vi "Robotics programming (Mohamed Elbakri 44171801).vi"() -> ()   [LabVIEW 2017]
uses:
  <vilib>/Native 3D Graph/xcontrol/3DPC_SurfacePlot.xctl
  <vilib>/Analysis/Matrix/Datatypes/RealMatrix.ctl
  <vilib>/Analysis/baseanly.llb/Real A x B.vi
  <vilib>/Analysis/baseanly.llb/Vector x A.vi
  <vilib>/Analysis/baseanly.llb/A x Vector.vi
  <vilib>/Analysis/NI_AALBase.lvlib
  <vilib>/Analysis/Matrix/NI_Matrix.lvlib
panel:
  in  "P2":dbl[](array[numeric])=[0.0, 0.0, 0.0]
  in  "P3":dbl[](array[numeric])=[0.0, 0.0, 0.0]
  in  "PE":dbl[](array[numeric])=[0.0, 0.0, 0.0]
  out "Out of range":bool
  out "?":dbl
  out "?":dbl
  out "PE":dbl[](array[numeric])
  out "P3":dbl[](array[numeric])
  out "P2":dbl[](array[numeric])
  out "b":dbl
  out "a":dbl
  out "T1":T1
  out "T2":T1
  out "T3":T1
  out "T1":T1
  out "T2":T1
  out "T3":T1
  out "T1":T1
  out "T2":T1
  out "T3":T1
  out "T1":T1
  out "T2":T1
  out "T3":T1
  in  "Z":dbl
  in  "Y":dbl
  in  "X":dbl
  in  "l0":dbl(slide) scale=0.0..10.0
  in  "l1":dbl(slide) scale=0.0..5.0
  in  "l2":dbl(slide) scale=0.0..5.0
  in  "l3":dbl(slide) scale=0.0..5.0
  out "Theta3":dbl(knob) scale=-90.0..90.0
  out "Theta2":dbl(knob) scale=-90.0..90.0
  out "Theta1":dbl(knob) scale=-180.0..180.0
  in  "Theta1":i16(knob) min=-180 max=180 step=1 scale=-180.0..180.0
  in  "Theta2":i8(knob) min=-90 max=90 step=1 scale=-90.0..90.0
  in  "Theta3":i8(knob) min=-90 max=90 step=1 scale=-90.0..90.0
  out "Control":dbl
  in  "Control":dbl=1.0 min=1.0 max=2.0 step=1.0
  out "S3":dbl(slide) scale=0.0..10.0
  out "S2":dbl(slide) scale=0.0..10.0
  out "S1":dbl(slide) scale=0.0..10.0
  in  "S3":i8(slide) scale=-10.0..10.0
  in  "S1":i8(slide) min=-10 max=10 step=1 scale=-10.0..10.0
  in  "S2":i8(slide) scale=-10.0..10.0
  in  "Robot":dbl=1.0 min=1.0 max=4.0 step=1.0 format="%#_4g"
  out "T3":T1
  out "T3":T1
  out "T3":T1
  out "T3":T1
  out "T1":T1
  out "T2":T1
  out "T1":T1
  out "T2":T1
  out "T1":T1
  out "T2":T1
  in  "stop":bool
  out "T2":T1
  out "T1":T1
  out "x_PE":dbl[](array[numeric])
  out "y_PE":dbl[](array[numeric])
  out "z_PE":dbl[](array[numeric])
  out "x_P3":dbl[](array[numeric])
  out "y_P3":dbl[](array[numeric])
  out "z_P3":dbl[](array[numeric])
  out "x_P2":dbl[](array[numeric])
  out "y_P2":dbl[](array[numeric])
  out "z_P2":dbl[](array[numeric])
  out "x_P1":dbl[](array[numeric])
  out "y_P1":dbl[](array[numeric])
  out "z_P1":dbl[](array[numeric])
  out "z_P0":dbl[](array[numeric])
  out "y_P0":dbl[](array[numeric])
  out "x_P0":dbl[](array[numeric])
  out "3D Graph":refnum<class "Base Datatype.lvclass">[](xcontrol)
  # "Robot Configuration"
  # "PE"
  # "Initial length"
  # "Joints position"
  # "L3"
  # "P3"
  # "L2"
  # "P2"
  # "L1"
  # "P1"
  # "L0"
  # "Control panel"
  # "Forward control"
  # "Joints control"
  # "Inverse control"
  # "Cartesian robot"
  # "Cylinderical robot"
  # "Spherical robot"
  # "Articulated robot"
  # "End-tip position"
  # "1: Cartesian robot"
  # "S3"
  # "L3"
  # "S3"
  # "2: Cylinderical robot"
  # "S3"
  # "Theta3"
  # "3: Spherical robot"
  # "L2"
  # "L2"
  # "4: Articulated robot"
  # "S2"
  # "Theta2"
  # "S2"
  # "Theta2"
  # "L1"
  # "L1"
  # "L1"
  # "Theta1"
  # "Theta1"
  # "S1"
  # "Theta1"
  # "1: Forward control"
  # "L0"
  # "L0"
  # "L0"
  # "2: Inverse control"
  # "L0"
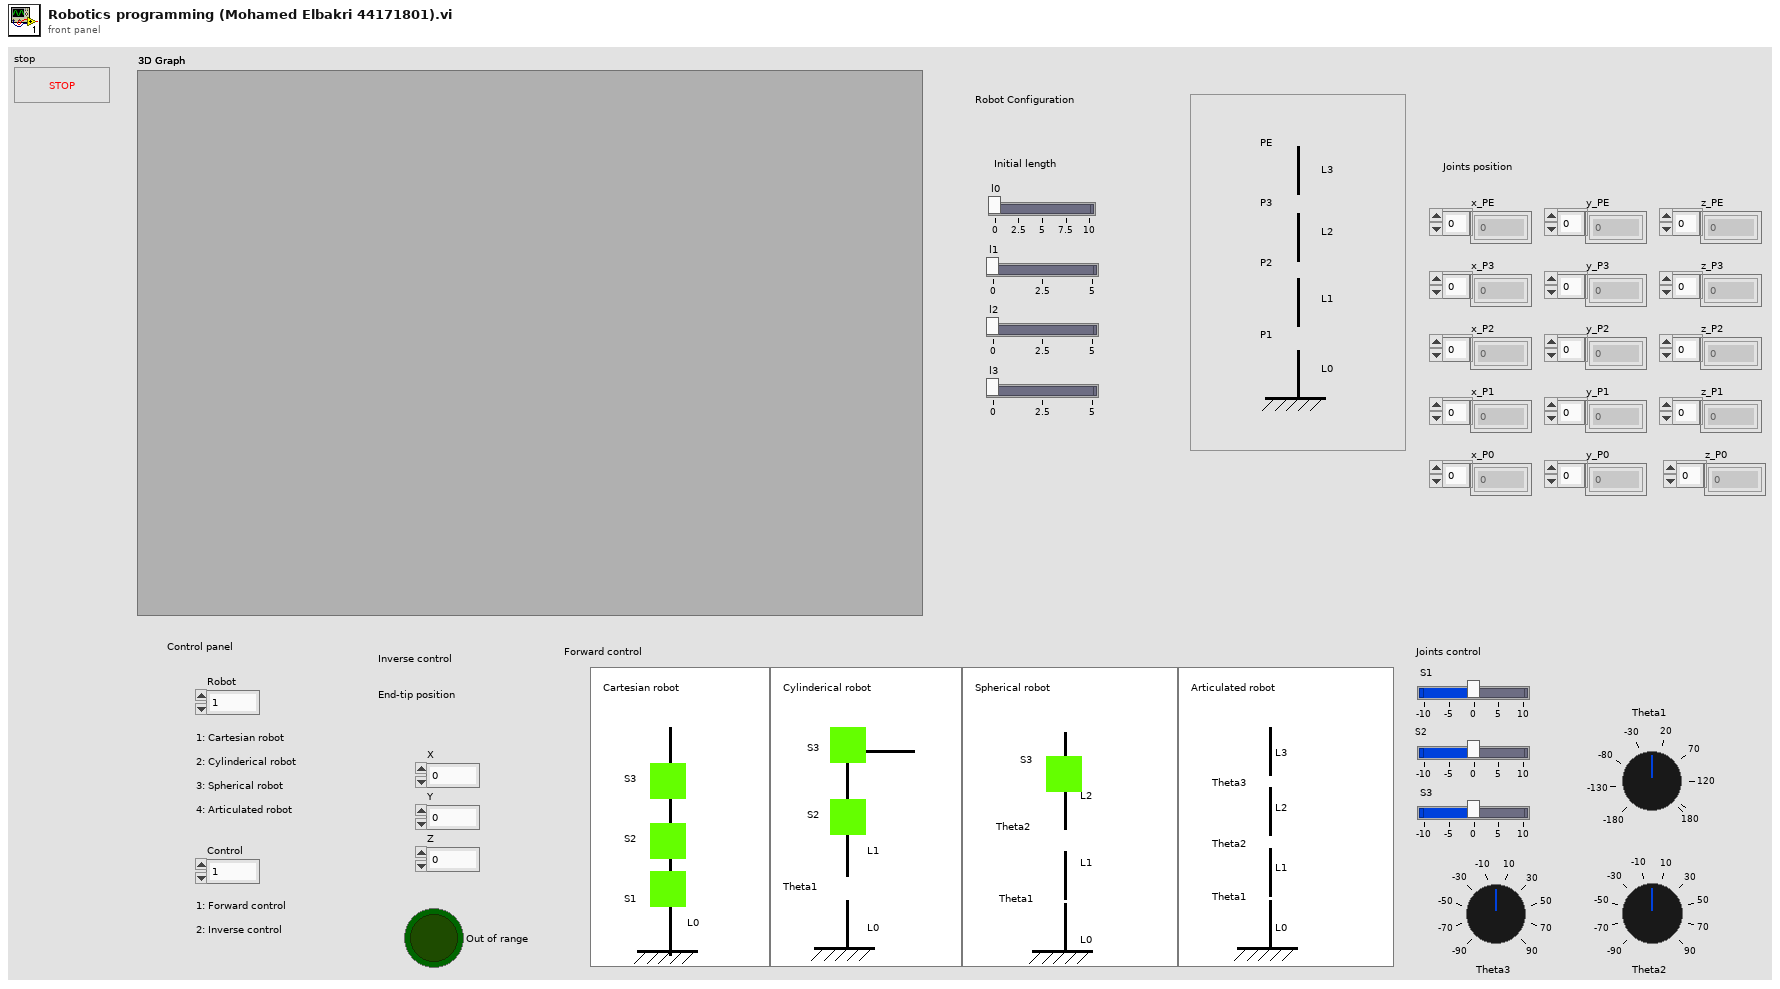
[diagram p1: front panel]
types:
  T1 = typedef "NI_Matrix.lvlib/RealMatrix.ctl" = dbl[][]
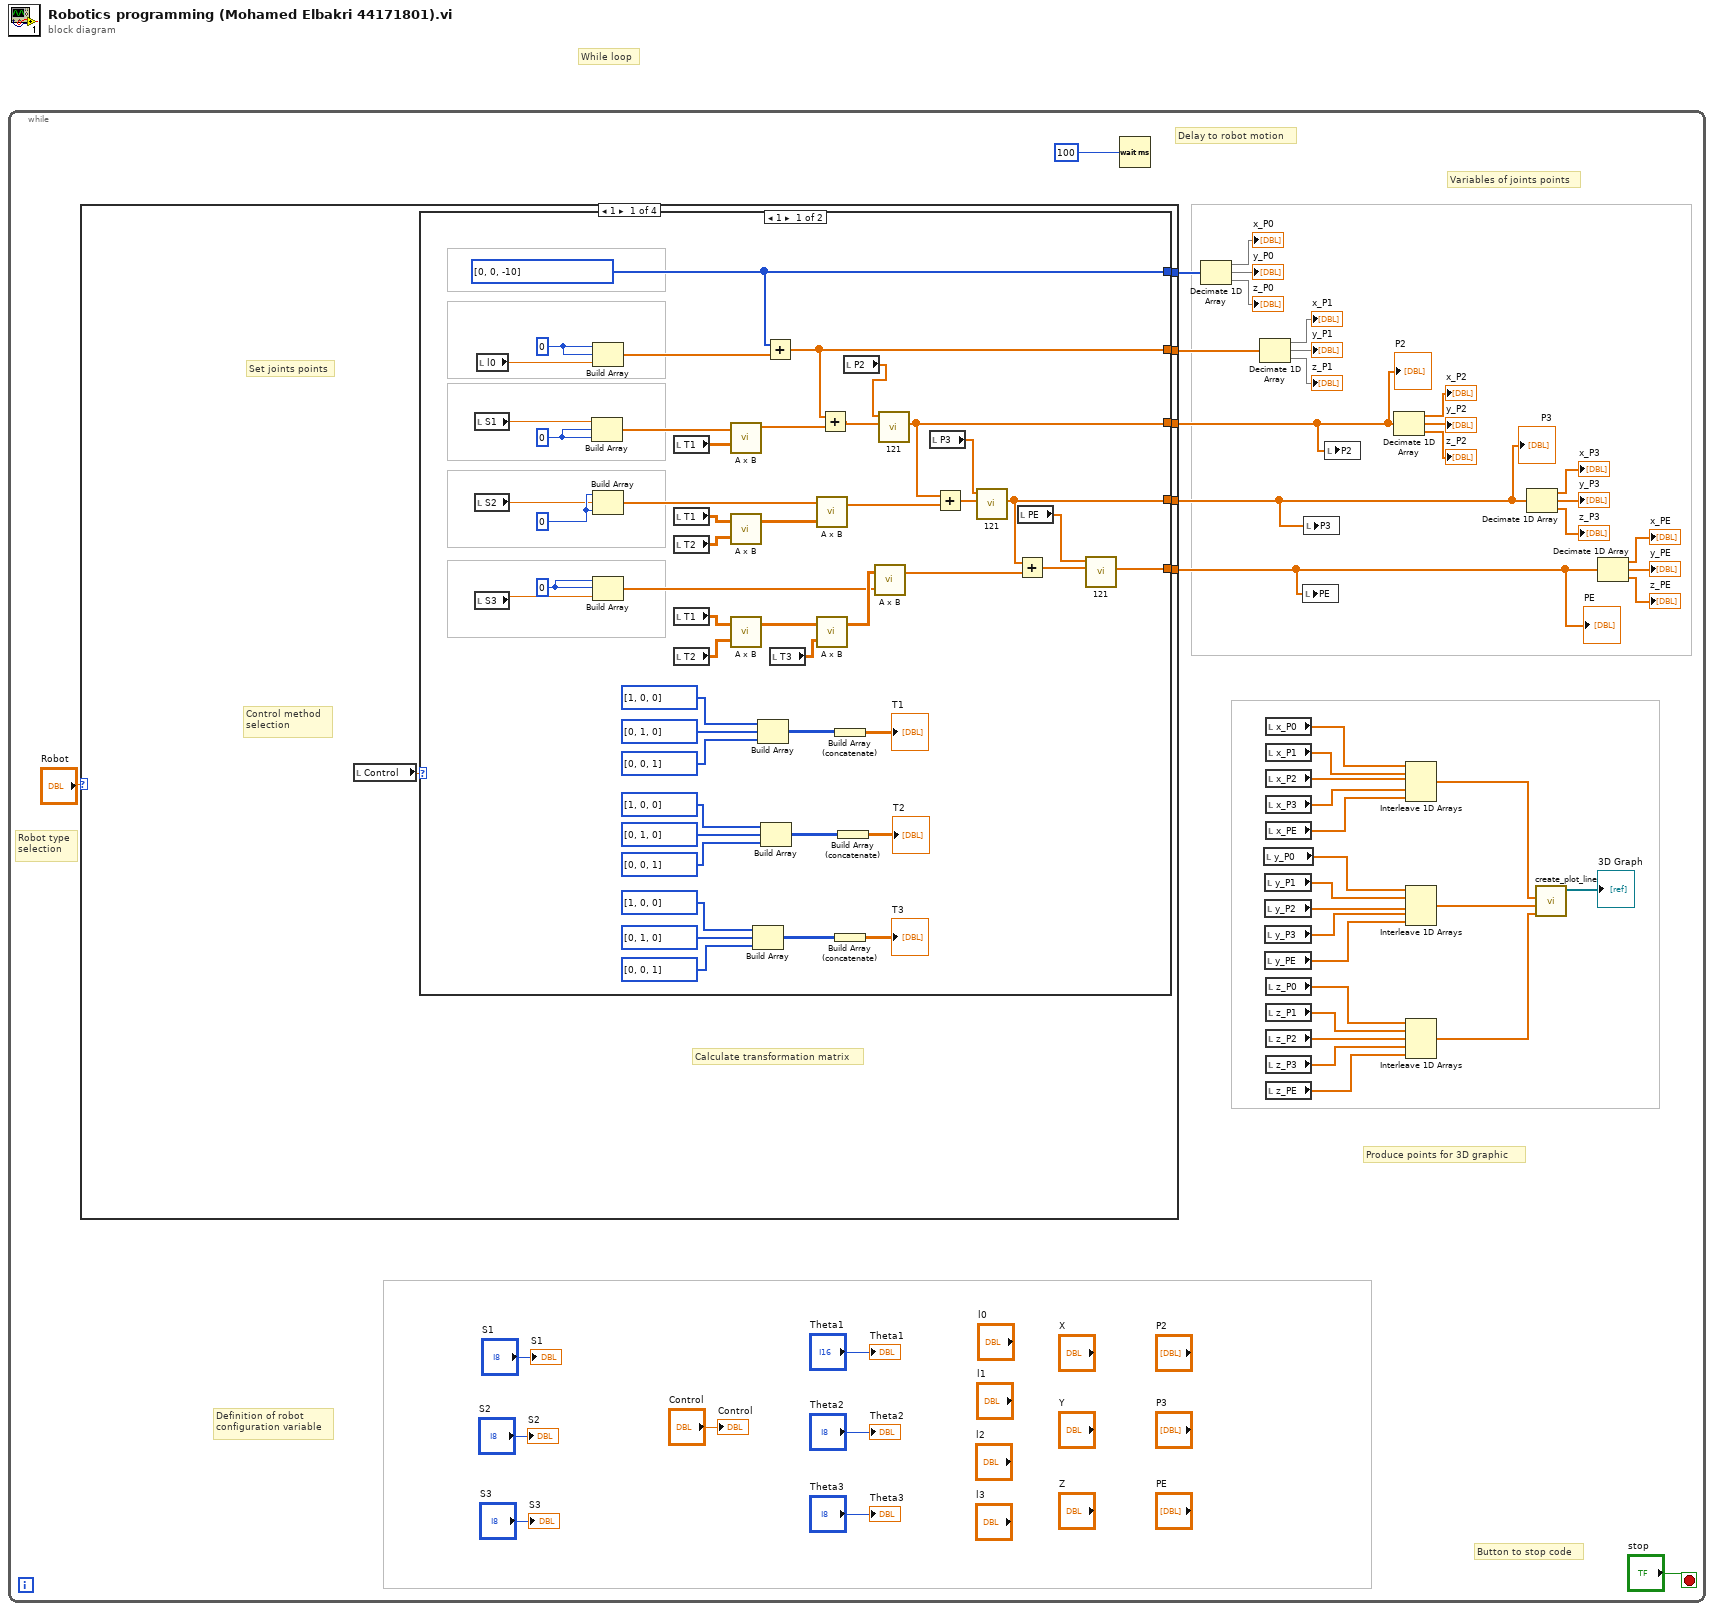
[diagram p0: block diagram]
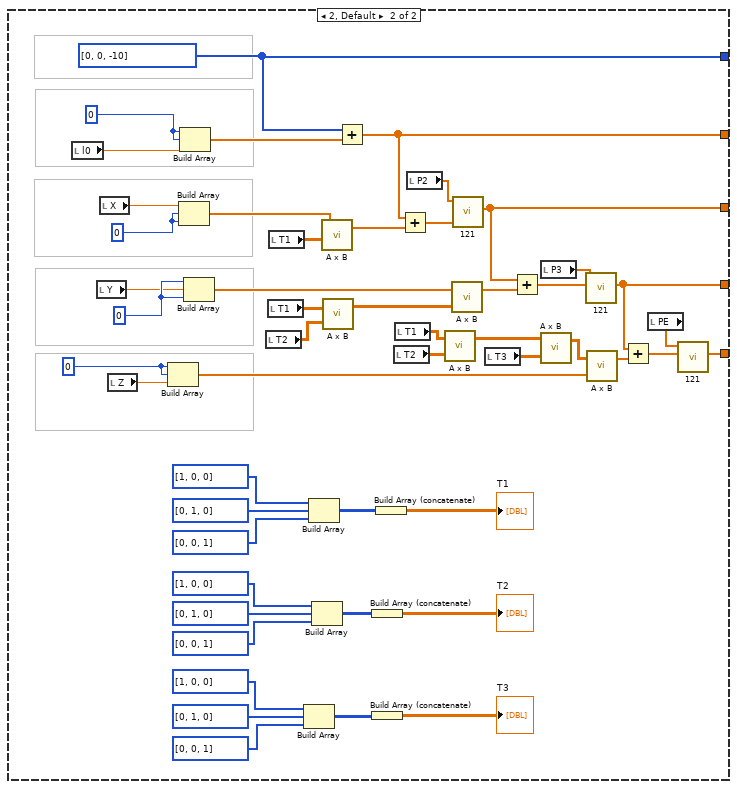
[diagram p2: hidden frame]
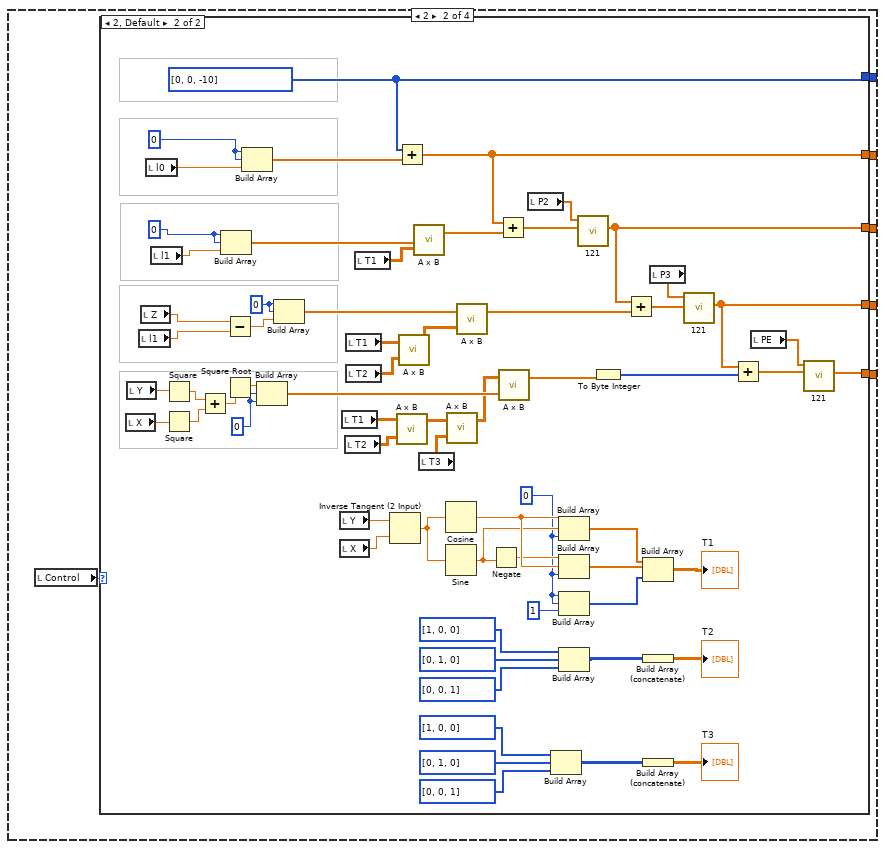
[diagram p3: hidden frame]
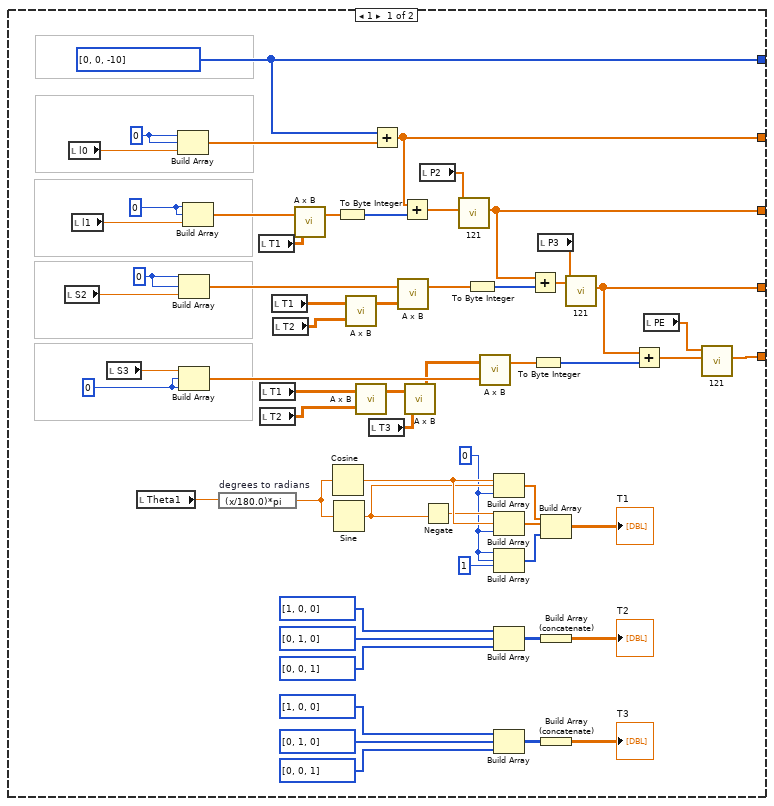
[diagram p4: hidden frame]
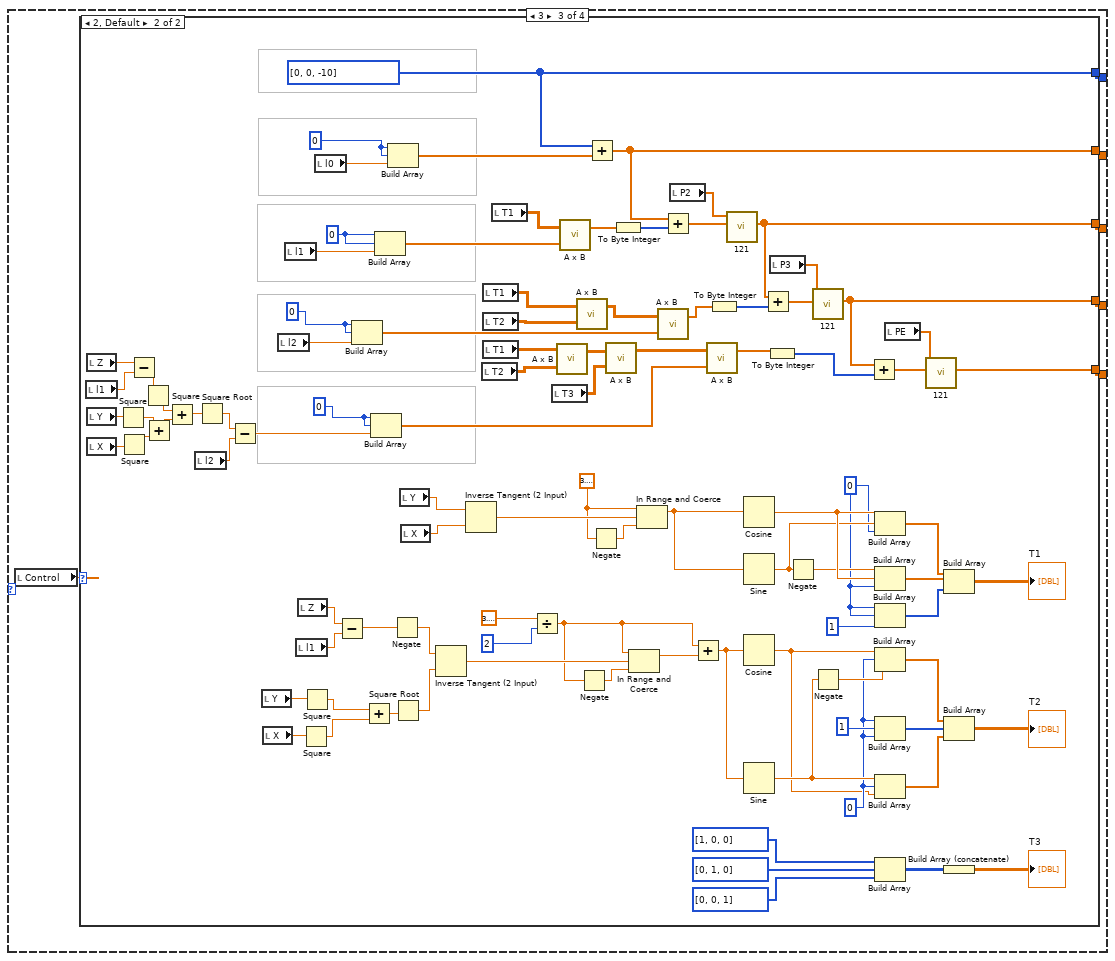
[diagram p5: hidden frame]
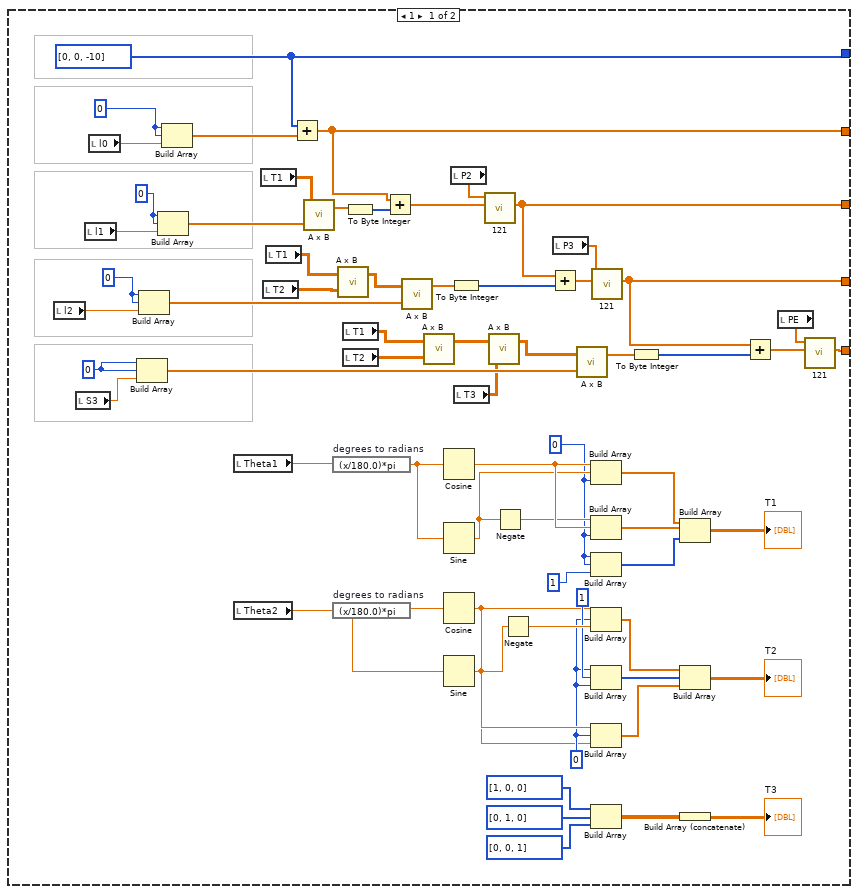
[diagram p6: hidden frame]
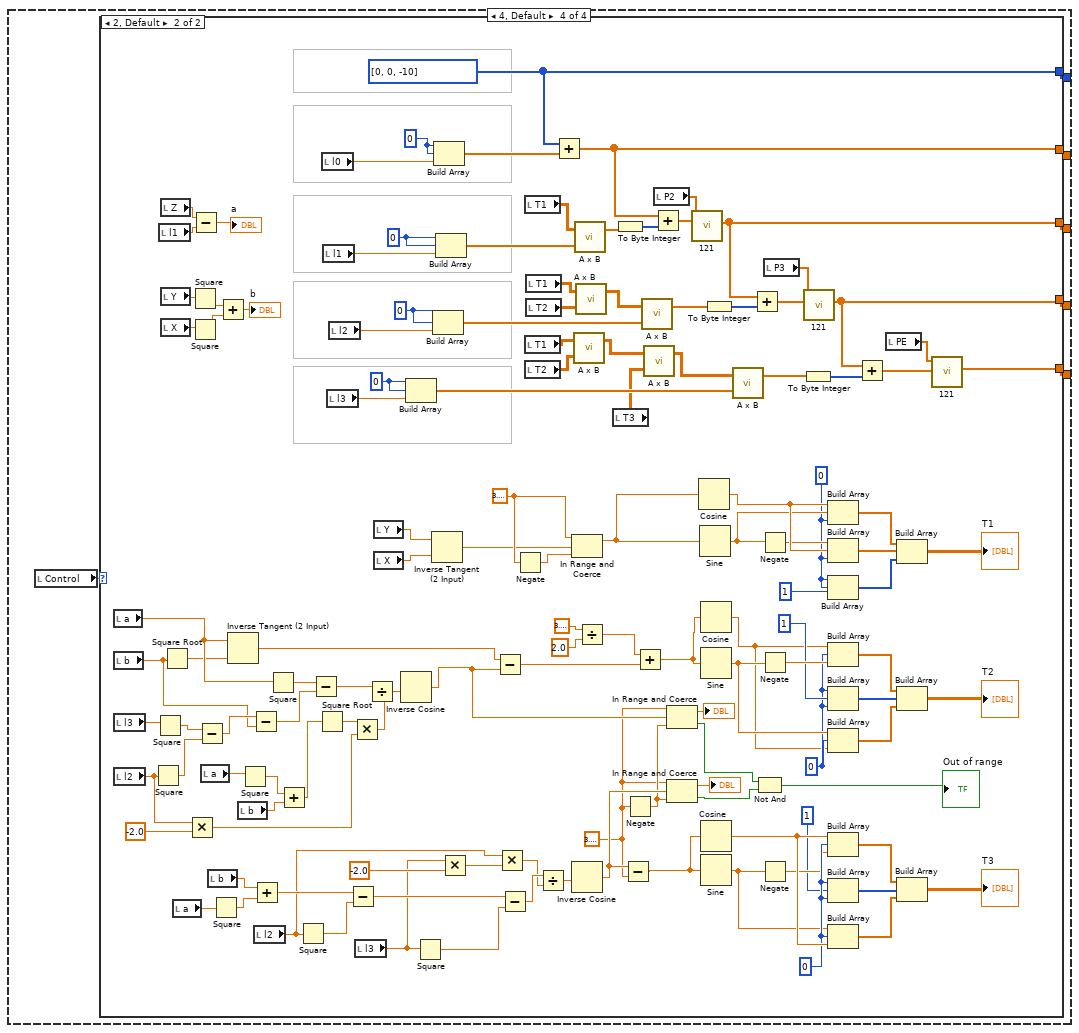
[diagram p7: hidden frame]
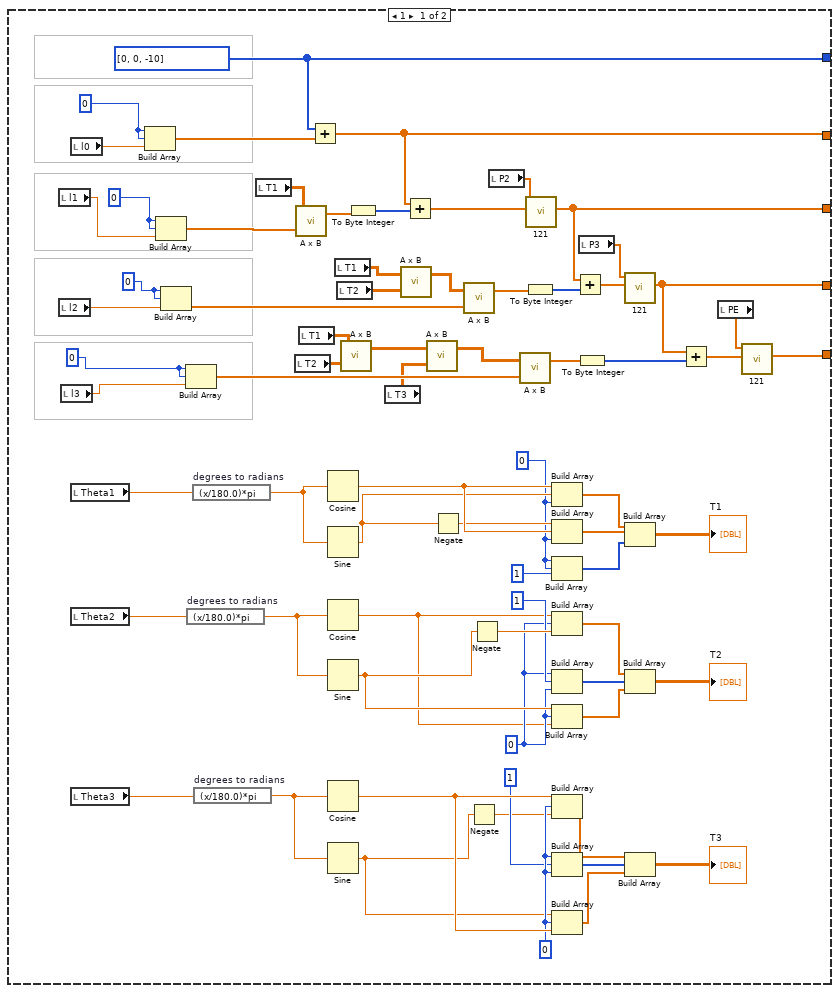
[diagram p8: hidden frame]
diagram:
  # "While loop"
  n1 = while {
    stop <- "stop" stop-if-true
    # "Delay to robot motion"
    # "Variables of joints points"
    # "Produce points for 3D graphic"
    # "Button to stop code"
    # "Robot type\nselection"
    # "Definition of robot\nconfiguration variable"
    n2 = case shown="1" "Robot" {
      tunnel: [w55 w161 w291 w458] -> w15
      tunnel: [w54 w160 w290 w457] -> w14
      tunnel: [w53 w159 w289 w456] -> w3
      tunnel: [w51 w158 w287 w454] -> w1
      tunnel: [w52 w157 w288 w455] -> w2
      frame 1 {
        # "Calculate transformation matrix"
        # "Set joints points"
        # "Control method\nselection"
        n3 = local read "Control"() -> (w50:dbl)
        n4 = case shown="1" w50 {
          tunnel: [w99 w149] -> w55
          tunnel: [w98 w128] -> w54
          tunnel: [w66 w125] -> w53
          tunnel: [w63 w120] -> w51
          tunnel: [w64 w123] -> w52
          frame 1 {
            w69 = 0
            w92 = 0
            w91 = 0
            w104 = 0
            w99 = i32[] [0, 0, -10]
            n5 = local read "S1"() -> (w68:dbl)
            n6 = local read "S2"() -> (w72:dbl)
            n7 = local read "S3"() -> (w60:dbl)
            n8 = local read "l0"() -> (w70:dbl)
            n9 = Build Array(w68, w92, w92) -> (w94:dbl[])
            n10 = Build Array(w69, w69, w70) -> (w71:dbl[])
            n11 = Build Array(w91, w72, w91) -> (w96:dbl[])
            n12 = Build Array(w104, w104, w60) -> (w59:dbl[])
            n13 = local read "T1"() -> (w93:T1)
            n14 = local read "T1"() -> (w103:T1)
            n15 = local read "T2"() -> (w102:T1)
            n16 = local read "T1"() -> (w101:T1)
            n17 = local read "T2"() -> (w100:T1)
            n18 = call-poly <vilib>:"A x B.vi"("Matrix A"=w93, "Vector V'"=w94) -> ("V' x A"=w61:dbl[])  [unwired: 1 out]
            n19 = call-poly <vilib>:"A x B.vi"("B"=w102, "A"=w103) -> ("A x B"=w95:T1)  [unwired: 1 out]
            n20 = call-poly <vilib>:"A x B.vi"("B"=w100, "A"=w101) -> ("A x B"=w90:T1)  [unwired: 1 out]
            n21 = Build Array(i32[] [1, 0, 0], i32[] [0, 1, 0], i32[] [0, 0, 1]) -> (w85:i32[][])
            n22 = Build Array(i32[] [1, 0, 0], i32[] [0, 1, 0], i32[] [0, 0, 1]) -> (w79:i32[][])
            n23 = Build Array(i32[] [1, 0, 0], i32[] [0, 1, 0], i32[] [0, 0, 1]) -> (w74:i32[][])
            n24 = Add(x=w99, y=w71) -> (x+y=w98:dbl[])
            n25 = local read "T3"() -> (w83:T1)
            n26 = call-poly <vilib>:"A x B.vi"("Matrix A"=w95, "Vector V'"=w96) -> ("V' x A"=w97:dbl[])  [unwired: 1 out]
            n27 = call-poly <vilib>:"A x B.vi"("B"=w83, "A"=w90) -> ("A x B"=w89:T1)  [unwired: 1 out]
            n28 = Add(x=w98, y=w61) -> (x+y=w67:dbl[])
            n29 = Build Array (concatenate)(w79) -> (→"T1":T1)
            n30 = Build Array (concatenate)(w85) -> (→"T3":T1)
            n31 = Build Array (concatenate)(w74) -> (→"T2":T1)
            n32 = local read "P2"() -> (w58:dbl[])
            n33 = call-poly <vilib>:"A x B.vi"("Vector"=w59, "A"=w89) -> ("A x Vector"=w105:dbl[])  [unwired: 1 out]
            n34 = call "121.vi"("V' x A"=w67, "Array in"=w58) -> ("interleaved array"=w66:dbl[])  [unwired: 9 in]
            n35 = local read "P3"() -> (w57:dbl[])
            n36 = Add(x=w66, y=w97) -> (x+y=w65:dbl[])
            n37 = call "121.vi"("V' x A"=w65, "Array in"=w57) -> ("interleaved array"=w64:dbl[])  [unwired: 9 in]
            n38 = Add(x=w64, y=w105) -> (x+y=w62:dbl[])
            n39 = local read "PE"() -> (w56:dbl[])
            n40 = call "121.vi"("V' x A"=w62, "Array in"=w56) -> ("interleaved array"=w63:dbl[])  [unwired: 9 in]
          }
          frame 2, Default {
            w131 = 0
            w141 = 0
            w140 = 0
            w154 = 0
            w149 = i32[] [0, 0, -10]
            n41 = local read "l0"() -> (w132:dbl)
            n42 = local read "Y"() -> (w129:dbl)
            n43 = local read "X"() -> (w130:dbl)
            n44 = local read "Z"() -> (w118:dbl)
            n45 = Build Array(w154, w154, w118) -> (w148:dbl[])
            n46 = Build Array(w130, w141, w141) -> (w143:dbl[])
            n47 = Build Array(w131, w131, w132) -> (w133:dbl[])
            n48 = Build Array(w140, w129, w140) -> (w146:dbl[])
            n49 = local read "T2"() -> (w152:T1)
            n50 = local read "T1"() -> (w153:T1)
            n51 = local read "T1"() -> (w142:T1)
            n52 = Build Array(i32[] [1, 0, 0], i32[] [0, 1, 0], i32[] [0, 0, 1]) -> (w106:i32[][])
            n53 = Build Array(i32[] [1, 0, 0], i32[] [0, 1, 0], i32[] [0, 0, 1]) -> (w108:i32[][])
            n54 = Build Array(i32[] [1, 0, 0], i32[] [0, 1, 0], i32[] [0, 0, 1]) -> (w107:i32[][])
            n55 = call-poly <vilib>:"A x B.vi"("Matrix A"=w142, "Vector V'"=w143) -> ("V' x A"=w144:dbl[])  [unwired: 1 out]
            n56 = call-poly <vilib>:"A x B.vi"("B"=w152, "A"=w153) -> ("A x B"=w145:T1)  [unwired: 1 out]
            n57 = Add(x=w149, y=w133) -> (x+y=w128:dbl[])
            n58 = Build Array (concatenate)(w107) -> (→"T2":T1)
            n59 = Build Array (concatenate)(w106) -> (→"T3":T1)
            n60 = Build Array (concatenate)(w108) -> (→"T1":T1)
            n61 = local read "T2"() -> (w150:T1)
            n62 = local read "T1"() -> (w151:T1)
            n63 = Add(x=w128, y=w144) -> (x+y=w126:dbl[])
            n64 = local read "P2"() -> (w127:dbl[])
            n65 = call-poly <vilib>:"A x B.vi"("B"=w150, "A"=w151) -> ("A x B"=w139:T1)  [unwired: 1 out]
            n66 = call-poly <vilib>:"A x B.vi"("Matrix A"=w145, "Vector V'"=w146) -> ("V' x A"=w147:dbl[])  [unwired: 1 out]
            n67 = call "121.vi"("V' x A"=w126, "Array in"=w127) -> ("interleaved array"=w125:dbl[])  [unwired: 9 in]
            n68 = local read "T3"() -> (w136:T1)
            n69 = Add(x=w125, y=w147) -> (x+y=w124:dbl[])
            n70 = local read "P3"() -> (w122:dbl[])
            n71 = call-poly <vilib>:"A x B.vi"("B"=w136, "A"=w139) -> ("A x B"=w138:T1)  [unwired: 1 out]
            n72 = call "121.vi"("V' x A"=w124, "Array in"=w122) -> ("interleaved array"=w123:dbl[])  [unwired: 9 in]
            n73 = call-poly <vilib>:"A x B.vi"("Vector"=w148, "A"=w138) -> ("A x Vector"=w155:dbl[])  [unwired: 1 out]
            n74 = Add(x=w123, y=w155) -> (x+y=w121:dbl[])
            n75 = local read "PE"() -> (w119:dbl[])
            n76 = call "121.vi"("V' x A"=w121, "Array in"=w119) -> ("interleaved array"=w120:dbl[])  [unwired: 9 in]
          }
        }
      }
      frame 2 {
        n77 = local read "Control"() -> (w156:dbl)
        n78 = case shown="2, Default" w156 {
          tunnel: [w182 w253] -> w161
          tunnel: [w203 w269] -> w160
          tunnel: [w181 w240] -> w159
          tunnel: [w176 w235] -> w158
          tunnel: [w178 w232] -> w157
          frame 1 {
            w182 = i32[] [0, 0, -10]
            w183 = 0
            w208 = 0
            w210 = 0
            w193 = 0
            w211 = 0
            n79 = local read "S2"() -> (w189:dbl)
            n80 = local read "l0"() -> (w185:dbl)
            n81 = local read "l1"() -> (w184:dbl)
            n82 = local read "S3"() -> (w188:dbl)
            n83 = local read "Theta1"() -> (w187:dbl)
            n84 = Build Array(w183, w183, w185) -> (w186:dbl[])
            n85 = Build Array(w208, w208, w189) -> (w200:dbl[])
            n86 = Build Array(w188, w193, w193) -> (w202:dbl[])
            n87 = Build Array(w211, w211, w184) -> (w197:dbl[])
            n88 = expression code="(x/180.0)*pi" "degrees to radians"(w187) -> (w220:dbl)
            n89 = local read "T1"() -> (w196:T1)
            n90 = local read "T1"() -> (w205:T1)
            n91 = local read "T2"() -> (w204:T1)
            n92 = local read "T1"() -> (w207:T1)
            n93 = local read "T2"() -> (w206:T1)
            n94 = call-poly <vilib>:"A x B.vi"("Matrix A"=w196, "Vector V'"=w197) -> ("V' x A"=w198:dbl[])  [unwired: 1 out]
            n95 = Cosine(x=w220) -> (cos(x)=w219:dbl)
            n96 = Sine(x=w220) -> (sin(x)=w218:dbl)
            n97 = To Byte Integer(number=w198) -> (8bit integer=w171:i8[])
            n98 = call-poly <vilib>:"A x B.vi"("B"=w206, "A"=w207) -> ("A x B"=w199:T1)  [unwired: 1 out]
            n99 = call-poly <vilib>:"A x B.vi"("B"=w204, "A"=w205) -> ("A x B"=w191:T1)  [unwired: 1 out]
            n100 = local read "T3"() -> (w192:T1)
            n101 = Add(x=w182, y=w186) -> (x+y=w203:dbl[])
            n102 = call-poly <vilib>:"A x B.vi"("Matrix A"=w199, "Vector V'"=w200) -> ("V' x A"=w201:dbl[])  [unwired: 1 out]
            n103 = Add(x=w203, y=w171) -> (x+y=w180:dbl[])
            n104 = call-poly <vilib>:"A x B.vi"("B"=w192, "A"=w191) -> ("A x B"=w190:T1)  [unwired: 1 out]
            n105 = local read "P2"() -> (w175:dbl[])
            n106 = Negate(x=w218) -> (-x=w217:dbl)
            n107 = call "121.vi"("V' x A"=w180, "Array in"=w175) -> ("interleaved array"=w181:dbl[])  [unwired: 9 in]
            n108 = To Byte Integer(number=w201) -> (8bit integer=w170:i8[])
            n109 = call-poly <vilib>:"A x B.vi"("Vector"=w202, "A"=w190) -> ("A x Vector"=w212:dbl[])  [unwired: 1 out]
            n110 = Build Array(w219, w218, w210) -> (w214:dbl[])
            n111 = Build Array(w217, w219, w210) -> (w215:dbl[])
            n112 = Build Array(w210, w210, 1) -> (w216:i32[])
            n113 = Build Array(i32[] [1, 0, 0], i32[] [0, 1, 0], i32[] [0, 0, 1]) -> (w168:i32[][])
            n114 = Build Array(i32[] [1, 0, 0], i32[] [0, 1, 0], i32[] [0, 0, 1]) -> (w169:i32[][])
            n115 = Add(x=w181, y=w170) -> (x+y=w179:dbl[])
            n116 = To Byte Integer(number=w212) -> (8bit integer=w172:i8[])
            n117 = local read "P3"() -> (w174:dbl[])
            n118 = Build Array(w214, w215, w216) -> (→"T1":T1)
            n119 = Build Array (concatenate)(w168) -> (→"T2":T1)
            n120 = Build Array (concatenate)(w169) -> (→"T3":T1)
            n121 = call "121.vi"("V' x A"=w179, "Array in"=w174) -> ("interleaved array"=w178:dbl[])  [unwired: 9 in]
            n122 = Add(x=w178, y=w172) -> (x+y=w177:dbl[])
            n123 = local read "PE"() -> (w173:dbl[])
            n124 = call "121.vi"("V' x A"=w177, "Array in"=w173) -> ("interleaved array"=w176:dbl[])  [unwired: 9 in]
          }
          frame 2, Default {
            w253 = i32[] [0, 0, -10]
            w254 = 0
            w274 = 0
            w276 = 0
            w260 = 0
            w277 = 0
            n125 = local read "X"() -> (w248:dbl)
            n126 = local read "Y"() -> (w249:dbl)
            n127 = local read "l1"() -> (w230:dbl)
            n128 = local read "Z"() -> (w251:dbl)
            n129 = local read "l0"() -> (w255:dbl)
            n130 = local read "l1"() -> (w250:dbl)
            n131 = Square(x=w249) -> (x^2=w247:dbl)
            n132 = Square(x=w248) -> (x^2=w246:dbl)
            n133 = Add(x=w247, y=w246) -> (x+y=w245:dbl)
            n134 = Build Array(w277, w277, w250) -> (w263:dbl[])
            n135 = Subtract(x=w251, y=w230) -> (x-y=w252:dbl)
            n136 = Square Root(x=w245) -> (sqrt(x)=w244:dbl)
            n137 = Build Array(w254, w254, w255) -> (w256:dbl[])
            n138 = Build Array(w244, w260, w260) -> (w268:dbl[])
            n139 = Build Array(w274, w274, w252) -> (w266:dbl[])
            n140 = local read "Y"() -> (w243:dbl)
            n141 = local read "X"() -> (w242:dbl)
            n142 = local read "T1"() -> (w271:T1)
            n143 = local read "T2"() -> (w270:T1)
            n144 = local read "T1"() -> (w273:T1)
            n145 = local read "T2"() -> (w272:T1)
            n146 = local read "T1"() -> (w262:T1)
            n147 = Inverse Tangent (2 Input)(1:w242, 2:w243) -> (0:w241:dbl)
            n148 = Add(x=w253, y=w256) -> (x+y=w269:dbl[])
            n149 = call-poly <vilib>:"A x B.vi"("B"=w270, "A"=w271) -> ("A x B"=w258:T1)  [unwired: 1 out]
            n150 = call-poly <vilib>:"A x B.vi"("B"=w272, "A"=w273) -> ("A x B"=w265:T1)  [unwired: 1 out]
            n151 = call-poly <vilib>:"A x B.vi"("Matrix A"=w262, "Vector V'"=w263) -> ("V' x A"=w264:dbl[])  [unwired: 1 out]
            n152 = local read "T3"() -> (w259:T1)
            n153 = Cosine(x=w241) -> (cos(x)=w285:dbl)
            n154 = Sine(x=w241) -> (sin(x)=w284:dbl)
            n155 = call-poly <vilib>:"A x B.vi"("B"=w259, "A"=w258) -> ("A x B"=w257:T1)  [unwired: 1 out]
            n156 = call-poly <vilib>:"A x B.vi"("Matrix A"=w265, "Vector V'"=w266) -> ("V' x A"=w267:dbl[])  [unwired: 1 out]
            n157 = Negate(x=w284) -> (-x=w283:dbl)
            n158 = Add(x=w269, y=w264) -> (x+y=w238:dbl[])
            n159 = call-poly <vilib>:"A x B.vi"("Vector"=w268, "A"=w257) -> ("A x Vector"=w278:dbl[])  [unwired: 1 out]
            n160 = local read "P2"() -> (w239:dbl[])
            n161 = Build Array(i32[] [1, 0, 0], i32[] [0, 1, 0], i32[] [0, 0, 1]) -> (w222:i32[][])
            n162 = Build Array(w285, w284, w276) -> (w280:dbl[])
            n163 = Build Array(w283, w285, w276) -> (w281:dbl[])
            n164 = Build Array(w276, w276, 1) -> (w282:i32[])
            n165 = Build Array(i32[] [1, 0, 0], i32[] [0, 1, 0], i32[] [0, 0, 1]) -> (w223:i32[][])
            n166 = call "121.vi"("V' x A"=w238, "Array in"=w239) -> ("interleaved array"=w240:dbl[])  [unwired: 9 in]
            n167 = To Byte Integer(number=w278) -> (8bit integer=w231:i8[])
            n168 = Add(x=w240, y=w267) -> (x+y=w237:dbl[])
            n169 = Build Array(w280, w281, w282) -> (→"T1":T1)
            n170 = Build Array (concatenate)(w223) -> (→"T2":T1)
            n171 = Build Array (concatenate)(w222) -> (→"T3":T1)
            n172 = local read "P3"() -> (w236:dbl[])
            n173 = call "121.vi"("V' x A"=w237, "Array in"=w236) -> ("interleaved array"=w232:dbl[])  [unwired: 9 in]
            n174 = Add(x=w232, y=w231) -> (x+y=w234:dbl[])
            n175 = local read "PE"() -> (w233:dbl[])
            n176 = call "121.vi"("V' x A"=w234, "Array in"=w233) -> ("interleaved array"=w235:dbl[])  [unwired: 9 in]
          }
        }
      }
      frame 3 {
        n177 = local read "Control"() -> (w286:dbl)
        n178 = case shown="2, Default" w286 {
          tunnel: [w313 w415] -> w291
          tunnel: [w329 w427] -> w290
          tunnel: [w306 w371] -> w289
          tunnel: [w300 w364] -> w287
          tunnel: [w303 w367] -> w288
          frame 1 {
            w313 = i32[] [0, 0, -10]
            w314 = 0
            w338 = 0
            w344 = 0
            w346 = 0
            w343 = 0
            w347 = 0
            n179 = local read "l2"() -> (w315:dbl)
            n180 = local read "S3"() -> (w321:dbl)
            n181 = local read "l1"() -> (w316:dbl)
            n182 = local read "l0"() -> (w317:dbl)
            n183 = Build Array(w343, w343, w321) -> (w327:dbl[])
            n184 = Build Array(w344, w344, w315) -> (w307:dbl[])
            n185 = Build Array(w347, w347, w316) -> (w312:dbl[])
            n186 = Build Array(w314, w314, w317) -> (w318:dbl[])
            n187 = local read "Theta1"() -> (w320:dbl)
            n188 = local read "Theta2"() -> (w319:dbl)
            n189 = local read "T1"() -> (w311:T1)
            n190 = local read "T2"() -> (w336:T1)
            n191 = local read "T1"() -> (w337:T1)
            n192 = Add(x=w313, y=w318) -> (x+y=w329:dbl[])
            n193 = call-poly <vilib>:"A x B.vi"("Vector"=w312, "A"=w311) -> ("A x Vector"=w310:dbl[])  [unwired: 1 out]
            n194 = expression code="(x/180.0)*pi" "degrees to radians"(w320) -> (w356:dbl)
            n195 = expression code="(x/180.0)*pi" "degrees to radians"(w319) -> (w342:dbl)
            n196 = call-poly <vilib>:"A x B.vi"("B"=w336, "A"=w337) -> ("A x B"=w308:T1)  [unwired: 1 out]
            n197 = local read "T1"() -> (w335:T1)
            n198 = local read "T2"() -> (w334:T1)
            n199 = To Byte Integer(number=w310) -> (8bit integer=w297:i8[])
            n200 = Add(x=w329, y=w297) -> (x+y=w305:dbl[])
            n201 = call-poly <vilib>:"A x B.vi"("Vector"=w307, "A"=w308) -> ("A x Vector"=w309:dbl[])  [unwired: 1 out]
            n202 = call-poly <vilib>:"A x B.vi"("B"=w334, "A"=w335) -> ("A x B"=w323:T1)  [unwired: 1 out]
            n203 = Cosine(x=w356) -> (cos(x)=w355:dbl)
            n204 = Sine(x=w356) -> (sin(x)=w354:dbl)
            n205 = Cosine(x=w342) -> (cos(x)=w328:dbl)
            n206 = Sine(x=w342) -> (sin(x)=w339:dbl)
            n207 = local read "P2"() -> (w304:dbl[])
            n208 = To Byte Integer(number=w309) -> (8bit integer=w296:i8[])
            n209 = local read "T3"() -> (w324:T1)
            n210 = call "121.vi"("V' x A"=w305, "Array in"=w304) -> ("interleaved array"=w306:dbl[])  [unwired: 9 in]
            n211 = call-poly <vilib>:"A x B.vi"("B"=w324, "A"=w323) -> ("A x B"=w322:T1)  [unwired: 1 out]
            n212 = Negate(x=w354) -> (-x=w353:dbl)
            n213 = Negate(x=w339) -> (-x=w341:dbl)
            n214 = Add(x=w306, y=w296) -> (x+y=w302:dbl[])
            n215 = local read "P3"() -> (w301:dbl[])
            n216 = call-poly <vilib>:"A x B.vi"("Vector"=w327, "A"=w322) -> ("A x Vector"=w348:dbl[])  [unwired: 1 out]
            n217 = Build Array(w355, w354, w346) -> (w350:dbl[])
            n218 = Build Array(w353, w355, w346) -> (w351:dbl[])
            n219 = Build Array(w346, w346, 1) -> (w352:i32[])
            n220 = Build Array(w328, w338, w341) -> (w333:dbl[])
            n221 = Build Array(w338, 1, w338) -> (w332:i32[])
            n222 = Build Array(w339, w338, w328) -> (w331:dbl[])
            n223 = Build Array(i32[] [1, 0, 0], i32[] [0, 1, 0], i32[] [0, 0, 1]) -> (w325:i32[][])
            n224 = call "121.vi"("V' x A"=w302, "Array in"=w301) -> ("interleaved array"=w303:dbl[])  [unwired: 9 in]
            n225 = To Byte Integer(number=w348) -> (8bit integer=w295:i8[])
            n226 = Build Array(w350, w351, w352) -> (→"T1":T1)
            n227 = Build Array(w333, w332, w331) -> (→"T2":T1)
            n228 = Build Array (concatenate)(w325) -> (→"T3":T1)
            n229 = Add(x=w303, y=w295) -> (x+y=w299:dbl[])
            n230 = local read "PE"() -> (w298:dbl[])
            n231 = call "121.vi"("V' x A"=w299, "Array in"=w298) -> ("interleaved array"=w300:dbl[])  [unwired: 9 in]
          }
          frame 2, Default {
            w378 = 3.141592653589793
            w415 = i32[] [0, 0, -10]
            w416 = 0
            w436 = 0
            w441 = 0
            w443 = 0
            w440 = 0
            w444 = 0
            n232 = local read "l1"() -> (w407:dbl)
            n233 = local read "Z"() -> (w408:dbl)
            n234 = local read "Y"() -> (w405:dbl)
            n235 = local read "X"() -> (w404:dbl)
            n236 = Square(x=w405) -> (x^2=w403:dbl)
            n237 = Square(x=w404) -> (x^2=w402:dbl)
            n238 = Subtract(x=w408, y=w407) -> (x-y=w397:dbl)
            n239 = Square(x=w397) -> (x^2=w406:dbl)
            n240 = Add(x=w403, y=w402) -> (x+y=w401:dbl)
            n241 = Add(x=w406, y=w401) -> (x+y=w400:dbl)
            n242 = local read "l2"() -> (w398:dbl)
            n243 = Square Root(x=w400) -> (sqrt(x)=w399:dbl)
            n244 = Subtract(x=w399, y=w398) -> (x-y=w396:dbl)
            n245 = local read "Y"() -> (w393:dbl)
            n246 = local read "X"() -> (w394:dbl)
            n247 = local read "l2"() -> (w417:dbl)
            n248 = local read "l1"() -> (w418:dbl)
            n249 = local read "l1"() -> (w395:dbl)
            n250 = local read "Z"() -> (w389:dbl)
            n251 = Square(x=w394) -> (x^2=w390:dbl)
            n252 = Square(x=w393) -> (x^2=w391:dbl)
            n253 = local read "l0"() -> (w419:dbl)
            n254 = Subtract(x=w389, y=w395) -> (x-y=w373:dbl)
            n255 = Build Array(w441, w441, w417) -> (w409:dbl[])
            n256 = Add(x=w391, y=w390) -> (x+y=w392:dbl)
            n257 = Build Array(w440, w440, w396) -> (w425:dbl[])
            n258 = Build Array(w444, w444, w418) -> (w414:dbl[])
            n259 = Build Array(w416, w416, w419) -> (w420:dbl[])
            n260 = Negate(x=w373) -> (-x=w374:dbl)
            n261 = Square Root(x=w392) -> (sqrt(x)=w386:dbl)
            n262 = local read "Y"() -> (w388:dbl)
            n263 = local read "X"() -> (w387:dbl)
            n264 = Inverse Tangent (2 Input)(1:w386, 2:w374) -> (0:w385:dbl)
            n265 = Inverse Tangent (2 Input)(1:w387, 2:w388) -> (0:w380:dbl)
            n266 = local read "T2"() -> (w432:T1)
            n267 = local read "T1"() -> (w435:T1)
            n268 = local read "T2"() -> (w434:T1)
            n269 = local read "T1"() -> (w433:T1)
            n270 = local read "T1"() -> (w413:T1)
            n271 = Divide(x=3.141592653589793, y=2) -> (x/y=w376:dbl)
            n272 = local read "T3"() -> (w423:T1)
            n273 = call-poly <vilib>:"A x B.vi"("B"=w432, "A"=w433) -> ("A x B"=w422:T1)  [unwired: 1 out]
            n274 = call-poly <vilib>:"A x B.vi"("Vector"=w414, "A"=w413) -> ("A x Vector"=w412:dbl[])  [unwired: 1 out]
            n275 = call-poly <vilib>:"A x B.vi"("B"=w434, "A"=w435) -> ("A x B"=w410:T1)  [unwired: 1 out]
            n276 = Negate(x=w376) -> (-x=w382:dbl)
            n277 = Add(x=w415, y=w420) -> (x+y=w427:dbl[])
            n278 = Negate(x=w378) -> (-x=w381:dbl)
            n279 = call-poly <vilib>:"A x B.vi"("B"=w423, "A"=w422) -> ("A x B"=w421:T1)  [unwired: 1 out]
            n280 = To Byte Integer(number=w412) -> (8bit integer=w363:i8[])
            n281 = In Range and Coerce(upper limit=w376, x=w385, lower limit=w382) -> (coerced(x)=w377:dbl)  [unwired: 1 out]
            n282 = In Range and Coerce(upper limit=w378, x=w380, lower limit=w381) -> (coerced(x)=w379:dbl)  [unwired: 1 out]
            n283 = call-poly <vilib>:"A x B.vi"("Vector"=w409, "A"=w410) -> ("A x Vector"=w411:dbl[])  [unwired: 1 out]
            n284 = Add(x=w427, y=w363) -> (x+y=w372:dbl[])
            n285 = local read "P2"() -> (w370:dbl[])
            n286 = Add(x=w376, y=w377) -> (x+y=w375:dbl)
            n287 = call-poly <vilib>:"A x B.vi"("Vector"=w425, "A"=w421) -> ("A x Vector"=w445:dbl[])  [unwired: 1 out]
            n288 = To Byte Integer(number=w411) -> (8bit integer=w362:i8[])
            n289 = call "121.vi"("V' x A"=w372, "Array in"=w370) -> ("interleaved array"=w371:dbl[])  [unwired: 9 in]
            n290 = Cosine(x=w379) -> (cos(x)=w452:dbl)
            n291 = Sine(x=w379) -> (sin(x)=w451:dbl)
            n292 = Cosine(x=w375) -> (cos(x)=w426:dbl)
            n293 = Sine(x=w375) -> (sin(x)=w437:dbl)
            n294 = Add(x=w371, y=w362) -> (x+y=w369:dbl[])
            n295 = To Byte Integer(number=w445) -> (8bit integer=w361:i8[])
            n296 = local read "P3"() -> (w368:dbl[])
            n297 = Negate(x=w451) -> (-x=w450:dbl)
            n298 = call "121.vi"("V' x A"=w369, "Array in"=w368) -> ("interleaved array"=w367:dbl[])  [unwired: 9 in]
            n299 = Negate(x=w437) -> (-x=w439:dbl)
            n300 = Add(x=w367, y=w361) -> (x+y=w366:dbl[])
            n301 = Build Array(w452, w451, w443) -> (w447:dbl[])
            n302 = Build Array(w450, w452, w443) -> (w448:dbl[])
            n303 = Build Array(w443, w443, 1) -> (w449:i32[])
            n304 = Build Array(w426, w436, w439) -> (w431:dbl[])
            n305 = Build Array(w436, 1, w436) -> (w430:i32[])
            n306 = Build Array(w437, w436, w426) -> (w429:dbl[])
            n307 = Build Array(i32[] [1, 0, 0], i32[] [0, 1, 0], i32[] [0, 0, 1]) -> (w360:i32[][])
            n308 = local read "PE"() -> (w365:dbl[])
            n309 = call "121.vi"("V' x A"=w366, "Array in"=w365) -> ("interleaved array"=w364:dbl[])  [unwired: 9 in]
            n310 = Build Array(w447, w448, w449) -> (→"T1":T1)
            n311 = Build Array(w431, w430, w429) -> (→"T2":T1)
            n312 = Build Array (concatenate)(w360) -> (→"T3":T1)
          }
        }
      }
      frame 4, Default {
        n313 = local read "Control"() -> (w453:dbl)
        n314 = case shown="2, Default" w453 {
          tunnel: [w478 w615] -> w458
          tunnel: [w503 w635] -> w457
          tunnel: [w469 w570] -> w456
          tunnel: [w464 w565] -> w454
          tunnel: [w466 w566] -> w455
          frame 1 {
            w478 = i32[] [0, 0, -10]
            w479 = 0
            w496 = 0
            w511 = 0
            w517 = 0
            w519 = 0
            w516 = 0
            w520 = 0
            n315 = local read "l1"() -> (w482:dbl)
            n316 = local read "l2"() -> (w481:dbl)
            n317 = local read "l3"() -> (w480:dbl)
            n318 = local read "l0"() -> (w483:dbl)
            n319 = local read "Theta1"() -> (w487:dbl)
            n320 = local read "Theta2"() -> (w486:dbl)
            n321 = local read "Theta3"() -> (w485:dbl)
            n322 = Build Array(w479, w479, w483) -> (w484:dbl[])
            n323 = Build Array(w520, w520, w482) -> (w476:dbl[])
            n324 = Build Array(w517, w517, w481) -> (w473:dbl[])
            n325 = Build Array(w516, w516, w480) -> (w501:dbl[])
            n326 = expression code="(x/180.0)*pi" "degrees to radians"(w486) -> (w515:dbl)
            n327 = expression code="(x/180.0)*pi" "degrees to radians"(w487) -> (w529:dbl)
            n328 = expression code="(x/180.0)*pi" "degrees to radians"(w485) -> (w492:dbl)
            n329 = local read "T1"() -> (w477:T1)
            n330 = local read "T2"() -> (w507:T1)
            n331 = call-poly <vilib>:"A x B.vi"("Vector"=w476, "A"=w477) -> ("A x Vector"=w475:dbl[])  [unwired: 1 out]
            n332 = local read "T1"() -> (w508:T1)
            n333 = Add(x=w478, y=w484) -> (x+y=w503:dbl[])
            n334 = Cosine(x=w529) -> (cos(x)=w528:dbl)
            n335 = Sine(x=w529) -> (sin(x)=w527:dbl)
            n336 = Cosine(x=w515) -> (cos(x)=w502:dbl)
            n337 = Sine(x=w515) -> (sin(x)=w512:dbl)
            n338 = Cosine(x=w492) -> (cos(x)=w500:dbl)
            n339 = Sine(x=w492) -> (sin(x)=w495:dbl)
            n340 = local read "T1"() -> (w510:T1)
            n341 = local read "T2"() -> (w509:T1)
            n342 = call-poly <vilib>:"A x B.vi"("B"=w507, "A"=w508) -> ("A x B"=w489:T1)  [unwired: 1 out]
            n343 = To Byte Integer(number=w475) -> (8bit integer=w462:i8[])
            n344 = local read "T3"() -> (w490:T1)
            n345 = call-poly <vilib>:"A x B.vi"("B"=w509, "A"=w510) -> ("A x B"=w474:T1)  [unwired: 1 out]
            n346 = Add(x=w503, y=w462) -> (x+y=w471:dbl[])
            n347 = call-poly <vilib>:"A x B.vi"("B"=w490, "A"=w489) -> ("A x B"=w488:T1)  [unwired: 1 out]
            n348 = Negate(x=w527) -> (-x=w526:dbl)
            n349 = call-poly <vilib>:"A x B.vi"("Vector"=w473, "A"=w474) -> ("A x Vector"=w472:dbl[])  [unwired: 1 out]
            n350 = Negate(x=w495) -> (-x=w493:dbl)
            n351 = Negate(x=w512) -> (-x=w514:dbl)
            n352 = local read "P2"() -> (w470:dbl[])
            n353 = call-poly <vilib>:"A x B.vi"("Vector"=w501, "A"=w488) -> ("A x Vector"=w521:dbl[])  [unwired: 1 out]
            n354 = To Byte Integer(number=w472) -> (8bit integer=w460:i8[])
            n355 = call "121.vi"("V' x A"=w471, "Array in"=w470) -> ("interleaved array"=w469:dbl[])  [unwired: 9 in]
            n356 = Build Array(w528, w527, w519) -> (w523:dbl[])
            n357 = Build Array(w526, w528, w519) -> (w524:dbl[])
            n358 = Build Array(w519, w519, 1) -> (w525:i32[])
            n359 = Build Array(w502, w511, w514) -> (w506:dbl[])
            n360 = Build Array(w511, 1, w511) -> (w505:i32[])
            n361 = Build Array(w512, w511, w502) -> (w504:dbl[])
            n362 = Build Array(w500, w496, w493) -> (w497:dbl[])
            n363 = Build Array(w496, 1, w496) -> (w498:i32[])
            n364 = Build Array(w495, w496, w500) -> (w499:dbl[])
            n365 = Add(x=w469, y=w460) -> (x+y=w468:dbl[])
            n366 = To Byte Integer(number=w521) -> (8bit integer=w461:i8[])
            n367 = local read "P3"() -> (w467:dbl[])
            n368 = call "121.vi"("V' x A"=w468, "Array in"=w467) -> ("interleaved array"=w466:dbl[])  [unwired: 9 in]
            n369 = Build Array(w523, w524, w525) -> (→"T1":T1)
            n370 = Build Array(w506, w505, w504) -> (→"T2":T1)
            n371 = Build Array(w497, w498, w499) -> (→"T3":T1)
            n372 = Add(x=w466, y=w461) -> (x+y=w465:dbl[])
            n373 = local read "PE"() -> (w463:dbl[])
            n374 = call "121.vi"("V' x A"=w465, "Array in"=w463) -> ("interleaved array"=w464:dbl[])  [unwired: 9 in]
          }
          frame 2, Default {
            w574 = 3.141592653589793
            w530 = 3.141592653589793 ("y")
            w615 = i32[] [0, 0, -10]
            w616 = 0
            w628 = 0
            w642 = 0
            w647 = 0
            w649 = 0
            w646 = 0
            w650 = 0
            n375 = local read "a"() -> (w554:dbl)
            n376 = local read "b"() -> (w595:dbl)
            n377 = local read "l3"() -> (w603:dbl)
            n378 = local read "l2"() -> (w593:dbl)
            n379 = Square(x=w593) -> (x^2=w601:dbl)
            n380 = Square(x=w603) -> (x^2=w602:dbl)
            n381 = local read "l1"() -> (w607:dbl)
            n382 = local read "Z"() -> (w608:dbl)
            n383 = local read "Y"() -> (w606:dbl)
            n384 = local read "X"() -> (w605:dbl)
            n385 = Square Root(x=w595) -> (sqrt(x)=w553:dbl)
            n386 = local read "a"() -> (w546:dbl)
            n387 = Multiply(x=w593, y=-2.0) -> (x*y=w594:dbl)
            n388 = Square(x=w606) -> (x^2=w597:dbl)
            n389 = Square(x=w605) -> (x^2=w604:dbl)
            n390 = Subtract(x=w608, y=w607) -> (x-y=→"a":dbl)
            n391 = Subtract(x=w602, y=w601) -> (x-y=w600:dbl)
            n392 = local read "a"() -> (w588:dbl)
            n393 = local read "b"() -> (w583:dbl)
            n394 = Square(x=w546) -> (x^2=w545:dbl)
            n395 = Add(x=w597, y=w604) -> (x+y=→"b":dbl)
            n396 = Inverse Tangent (2 Input)(1:w553, 2:w554) -> (0:w549:dbl)
            n397 = local read "b"() -> (w586:dbl)
            n398 = Square(x=w588) -> (x^2=w587:dbl)
            n399 = Subtract(x=w600, y=w595) -> (x-y=w599:dbl)
            n400 = Add(x=w583, y=w545) -> (x+y=w582:dbl)
            n401 = local read "l2"() -> (w547:dbl)
            n402 = Square(x=w554) -> (x^2=w598:dbl)
            n403 = Add(x=w587, y=w586) -> (x+y=w584:dbl)
            n404 = Square(x=w547) -> (x^2=w577:dbl)
            n405 = Subtract(x=w598, y=w599) -> (x-y=w590:dbl)
            n406 = Square Root(x=w584) -> (sqrt(x)=w585:dbl)
            n407 = local read "l0"() -> (w620:dbl)
            n408 = local read "l1"() -> (w619:dbl)
            n409 = local read "l3"() -> (w617:dbl)
            n410 = local read "l2"() -> (w618:dbl)
            n411 = Subtract(x=w582, y=w577) -> (x-y=w581:dbl)
            n412 = Multiply(x=w585, y=w594) -> (x*y=w589:dbl)
            n413 = local read "l3"() -> (w548:dbl)
            n414 = Divide(x=w590, y=w589) -> (x/y=w591:dbl)
            n415 = local read "Y"() -> (w556:dbl)
            n416 = local read "X"() -> (w555:dbl)
            n417 = Inverse Cosine(1:w591) -> (0:w535:dbl)
            n418 = Build Array(w646, w646, w617) -> (w633:dbl[])
            n419 = Square(x=w548) -> (x^2=w576:dbl)
            n420 = Inverse Tangent (2 Input)(1:w555, 2:w556) -> (0:w557:dbl)
            n421 = Build Array(w647, w647, w618) -> (w610:dbl[])
            n422 = Build Array(w616, w616, w620) -> (w621:dbl[])
            n423 = Build Array(w650, w650, w619) -> (w613:dbl[])
            n424 = Multiply(x=w548, y=-2.0) -> (x*y=w578:dbl)
            n425 = Subtract(x=w549, y=w535) -> (x-y=w540:dbl)
            n426 = Multiply(x=w547, y=w578) -> (x*y=w575:dbl)
            n427 = Subtract(x=w581, y=w576) -> (x-y=w580:dbl)
            n428 = Negate(x=w574) -> (-x=w539:dbl)
            n429 = local read "T1"() -> (w614:T1)
            n430 = local read "T1"() -> (w641:T1)
            n431 = local read "T2"() -> (w640:T1)
            n432 = local read "T1"() -> (w558:T1)
            n433 = local read "T2"() -> (w559:T1)
            n434 = Divide(x=w580, y=w575) -> (x/y=w572:dbl)
            n435 = Add(x=w615, y=w621) -> (x+y=w635:dbl[])
            n436 = In Range and Coerce(upper limit=w574, x=w557, lower limit=w539) -> (coerced(x)=w573:dbl)  [unwired: 1 out]
            n437 = Inverse Cosine(1:w572) -> (0:w537:dbl)
            n438 = call-poly <vilib>:"A x B.vi"("B"=w640, "A"=w641) -> ("A x B"=w623:T1)  [unwired: 1 out]
            n439 = call-poly <vilib>:"A x B.vi"("Vector"=w613, "A"=w614) -> ("A x Vector"=w612:dbl[])  [unwired: 1 out]
            n440 = call-poly <vilib>:"A x B.vi"("B"=w559, "A"=w558) -> ("A x B"=w611:T1)  [unwired: 1 out]
            n441 = Divide(x=3.141592653589793, y=2.0) -> (x/y=w538:dbl)
            n442 = local read "T3"() -> (w624:T1)
            n443 = To Byte Integer(number=w612) -> (8bit integer=w562:i8[])
            n444 = Subtract(x=w537, y=w530) -> (x-y=w544:dbl)
            n445 = Negate(x=w530) -> (-x=w531:dbl)
            n446 = Add(x=w538, y=w540) -> (x+y=w543:dbl)
            n447 = call-poly <vilib>:"A x B.vi"("Vector"=w610, "A"=w611) -> ("A x Vector"=w609:dbl[])  [unwired: 1 out]
            n448 = call-poly <vilib>:"A x B.vi"("B"=w624, "A"=w623) -> ("A x B"=w622:T1)  [unwired: 1 out]
            n449 = Add(x=w635, y=w562) -> (x+y=w571:dbl[])
            n450 = local read "P2"() -> (w569:dbl[])
            n451 = In Range and Coerce(upper limit=w530, x=w535, lower limit=w531) -> (coerced(x)=→"?":dbl, In Range?=w533:bool)
            n452 = In Range and Coerce(upper limit=w530, x=w537, lower limit=w531) -> (coerced(x)=→"?":dbl, In Range?=w534:bool)
            n453 = call "121.vi"("V' x A"=w571, "Array in"=w569) -> ("interleaved array"=w570:dbl[])  [unwired: 9 in]
            n454 = Cosine(x=w573) -> (cos(x)=w658:dbl)
            n455 = Sine(x=w573) -> (sin(x)=w657:dbl)
            n456 = Cosine(x=w543) -> (cos(x)=w634:dbl)
            n457 = Sine(x=w543) -> (sin(x)=w643:dbl)
            n458 = Cosine(x=w544) -> (cos(x)=w632:dbl)
            n459 = Sine(x=w544) -> (sin(x)=w627:dbl)
            n460 = To Byte Integer(number=w609) -> (8bit integer=w561:i8[])
            n461 = call-poly <vilib>:"A x B.vi"("Vector"=w633, "A"=w622) -> ("A x Vector"=w651:dbl[])  [unwired: 1 out]
            n462 = Add(x=w570, y=w561) -> (x+y=w568:dbl[])
            n463 = Not And(1:w534, 2:w533) -> (0:→"Out of range":bool)
            n464 = Negate(x=w657) -> (-x=w656:dbl)
            n465 = Negate(x=w643) -> (-x=w645:dbl)
            n466 = Negate(x=w627) -> (-x=w626:dbl)
            n467 = local read "P3"() -> (w567:dbl[])
            n468 = To Byte Integer(number=w651) -> (8bit integer=w560:i8[])
            n469 = call "121.vi"("V' x A"=w568, "Array in"=w567) -> ("interleaved array"=w566:dbl[])  [unwired: 9 in]
            n470 = Build Array(w658, w657, w649) -> (w653:dbl[])
            n471 = Build Array(w656, w658, w649) -> (w654:dbl[])
            n472 = Build Array(w649, w649, 1) -> (w655:i32[])
            n473 = Build Array(w634, w642, w645) -> (w639:dbl[])
            n474 = Build Array(w642, 1, w642) -> (w638:i32[])
            n475 = Build Array(w643, w642, w634) -> (w637:dbl[])
            n476 = Build Array(w632, w628, w626) -> (w629:dbl[])
            n477 = Build Array(w628, 1, w628) -> (w630:i32[])
            n478 = Build Array(w627, w628, w632) -> (w631:dbl[])
            n479 = Add(x=w566, y=w560) -> (x+y=w564:dbl[])
            n480 = local read "PE"() -> (w563:dbl[])
            n481 = Build Array(w653, w654, w655) -> (→"T1":T1)
            n482 = Build Array(w639, w638, w637) -> (→"T2":T1)
            n483 = Build Array(w629, w630, w631) -> (→"T3":T1)
            n484 = call "121.vi"("V' x A"=w564, "Array in"=w563) -> ("interleaved array"=w565:dbl[])  [unwired: 9 in]
          }
        }
      }
    }
    "P2" <- w3
    "P3" <- w2
    "PE" <- w1
    n485 = Wait (ms)(milliseconds to wait=u32 100) -> ()  [unwired: 1 out]
    n486 = Decimate 1D Array(w15) -> (→"x_P0":i32[], →"y_P0":i32[], →"z_P0":i32[])
    n487 = Decimate 1D Array(w14) -> (→"x_P1":dbl[], →"y_P1":dbl[], →"z_P1":dbl[])
    n488 = local read "y_P0"() -> (w25:dbl[])
    n489 = local read "y_P1"() -> (w26:dbl[])
    n490 = local read "y_P2"() -> (w27:dbl[])
    n491 = local read "y_P3"() -> (w28:dbl[])
    n492 = local read "y_PE"() -> (w29:dbl[])
    n493 = local read "x_P0"() -> (w34:dbl[])
    n494 = local read "x_P1"() -> (w33:dbl[])
    n495 = local read "x_P2"() -> (w32:dbl[])
    n496 = local read "x_P3"() -> (w31:dbl[])
    n497 = local read "x_PE"() -> (w30:dbl[])
    n498 = local read "z_P0"() -> (w24:dbl[])
    n499 = local read "z_P1"() -> (w23:dbl[])
    n500 = local read "z_P2"() -> (w22:dbl[])
    n501 = local read "z_P3"() -> (w21:dbl[])
    n502 = local read "z_PE"() -> (w20:dbl[])
    n503 = local write "PE"(w1) -> ()
    n504 = local write "P3"(w2) -> ()
    n505 = local write "P2"(w3) -> ()
    n506 = Decimate 1D Array(w3) -> (→"x_P2":dbl[], →"y_P2":dbl[], →"z_P2":dbl[])
    n507 = Interleave 1D Arrays(w34, w33, w32, w31, w30) -> (w18:dbl[])
    n508 = Interleave 1D Arrays(w25, w26, w27, w28, w29) -> (w17:dbl[])
    n509 = Interleave 1D Arrays(w24, w23, w22, w21, w20) -> (w16:dbl[])
    n510 = Decimate 1D Array(w2) -> (→"x_P3":dbl[], →"y_P3":dbl[], →"z_P3":dbl[])
    n511 = call <vilib>:"create_plot_line.vi"("z vector"=w16, "y vector"=w17, "x vector"=w18) -> ("plots out"=→"3D Graph":refnum<class "Base Datatype.lvclass">[])  [unwired: 2 in, 6 out]
    n512 = Decimate 1D Array(w1) -> (→"x_PE":dbl[], →"y_PE":dbl[], →"z_PE":dbl[])
    "S1" <- "S1"
    "S2" <- "S2"
    "S3" <- "S3"
    "Control" <- "Control"
    "Theta1" <- "Theta1"
    "Theta2" <- "Theta2"
    "Theta3" <- "Theta3"
  }
